vi "Config.vi"(8 "error in (no error)":errorcluster, 9 "Channel Name":string, 10 "Setting":T1={"Max. Volt"=10.0, "Current Limit"=0.5, "Measurement Type"=1, "Voltage Level"=10.0} {"Measurement Type" items=["Voltage"=1, "Current"=0]}, 11 "Keysight 6700C in":refnum<class "Keysight 6700C.lvclass">) -> (0 "error out":errorcluster, 3 "Keysight 6700C out":refnum<class "Keysight 6700C.lvclass">)   [LabVIEW 2021, in "Concrete.lvlib" / "Keysight 6700C.lvclass"]
uses:
  Keysight 6700C.lvclass
  Keysight 6700C.lvclass/Keysight 6700C.ctl
  <instrlib>/Agilent N6700 Series/Agilent N6700 Series.lvlib
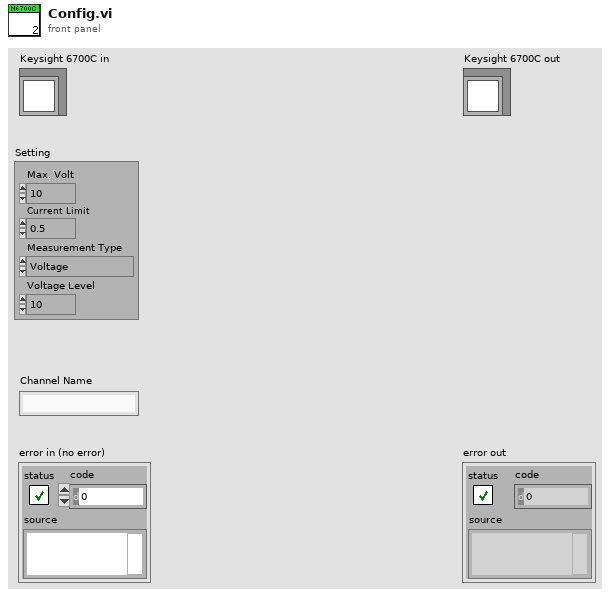
[diagram p1: front panel]
types:
  T1 = cluster{"Max. Volt":dbl, "Current Limit":dbl, "Measurement Type":i32, "Voltage Level":dbl}
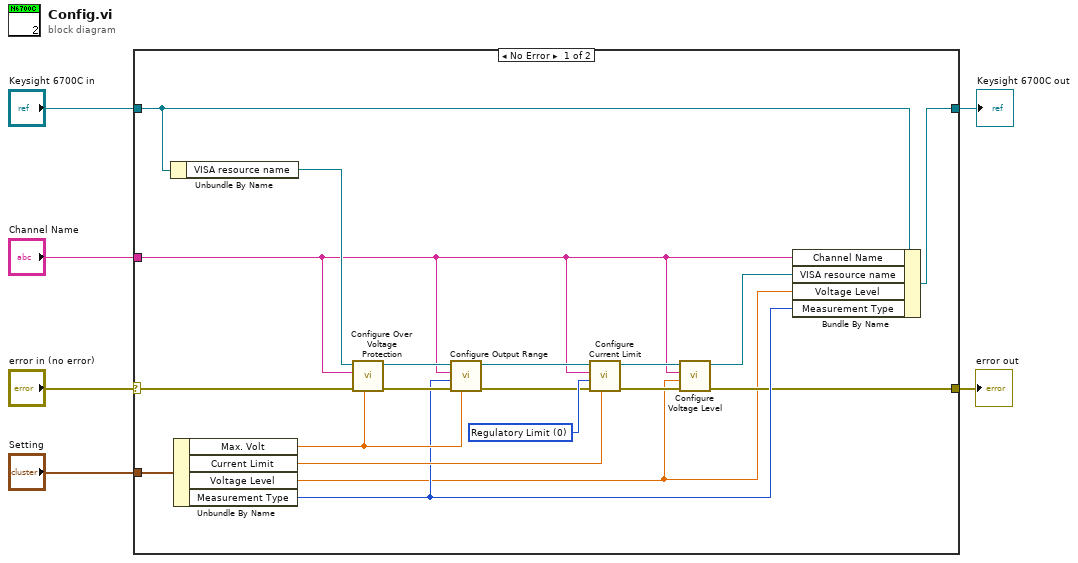
[diagram p0: block diagram]
diagram:
  n1 = case shown="No Error" "error in (no error)" {
    selector: "error in (no error)" -> [w21 w27]
    tunnel: [w9 w27] -> w5
    tunnel: [w22 w26] -> w3
    tunnel: "Keysight 6700C in" -> [w23 w26]
    tunnel: "Setting" -> [w24 _]
    tunnel: "Channel Name" -> [w10 _]
    frame No Error {
      w25 = 0 items=["Regulatory Limit", "Trip Limit"] ("Behavior (0: Regulatory Limit)")
      n2 = Unbundle By Name(w23) -> ("VISA resource name"=w20:refnum<visa-resource-name>)
      n3 = Unbundle By Name(w24) -> ("Max. Volt"=w17:dbl, "Current Limit"=w16:dbl, "Voltage Level"=w8:dbl, "Measurement Type"=w15:i32)
      n4 = call <instrlib>:"Configure Over Voltage Protection.vi"("Limit (0.0 volts)"=w17, "error in (no error)"=w21, "Channel Name (1)"=w10, "VISA resource name"=w20) -> ("error out"=w19:errorcluster, "VISA resource name out"=w18:refnum<visa-resource-name>)  [unwired: 6 in]
      n5 = call <instrlib>:"Configure Output Range.vi"("Range (0.0)"=w17, "error in (no error)"=w19, "Range Type (1: Voltage)"=w15, "Channel Name (1)"=w10, "VISA resource name"=w18) -> ("error out"=w14:errorcluster, "VISA resource name out"=w13:refnum<visa-resource-name>)  [unwired: 5 in]
      n6 = call <instrlib>:"Configure Current Limit.vi"("Limit (0.0 amps)"=w16, "error in (no error)"=w14, "Behavior (0: Regulatory Limit)"=w25, "Channel Name (1)"=w10, "VISA resource name"=w13) -> ("error out"=w12:errorcluster, "VISA resource name out"=w11:refnum<visa-resource-name>)  [unwired: 5 in]
      n7 = call <instrlib>:"Configure Voltage Level.vi"("error in (no error)"=w12, "Level  (0.0 volts)"=w8, "Channel Name (1)"=w10, "VISA resource name"=w11) -> ("error out"=w9:errorcluster, "VISA resource name out"=w7:refnum<visa-resource-name>)  [unwired: 6 in]
      n8 = Bundle By Name(cluster=w23, "Channel Name"=w10, "VISA resource name"=w7, "Voltage Level"=w8, "Measurement Type"=w15) -> (w22:refnum<class "Keysight 6700C.lvclass">)
    }
    frame Error {
    }
  }
  "error out" <- w5
  "Keysight 6700C out" <- w3
